vi "Team Member's Favorite Color.vi"(11 "Team Member Name":string) -> (0 "error out":errorcluster, 3 "Favorite Color":u32(colorbox))   [LabVIEW 2024]
uses:
  Team Member/Team Member.lvclass
panel:
  # "Specify your name (i.e. the name of your class) and run the VI. Your favorite color should be displayed."
  # "Note: This VI should require no modification in order to display your favorite color."
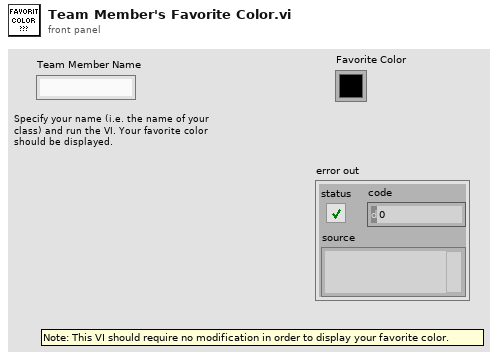
[diagram p1: front panel]
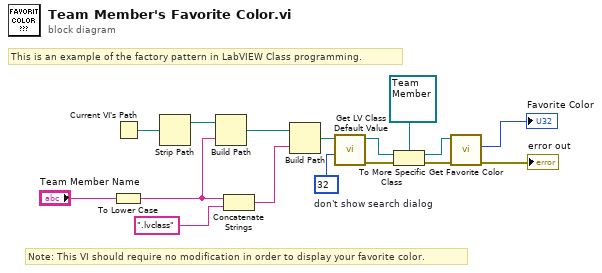
[diagram p0: block diagram]
diagram:
  w1 = u32 32  # don't show search dialog
  # "This is an example of the factory pattern in LabVIEW Class programming."
  # "Note: This VI should require no modification in order to display your favorite color."
  n1 = To Lower Case(string="Team Member Name") -> (all lower case string=w2:string)
  n2 = Current VI's Path() -> (path=w9:path)
  n3 = Strip Path(path=w9) -> (stripped path=w8:path)  [unwired: 1 out]
  n4 = Build Path(base path=w8, name or relative path=w2) -> (appended path=w6:path)
  n5 = Concatenate Strings(w2, ".lvclass" ("string")) -> (w3:string)
  n6 = Build Path(base path=w6, name or relative path=w3) -> (appended path=w7:path)
  n7 = call <vilib>:"Get LV Class Default Value.vi"("options"=w1, "class path"=w7) -> ("error out"=w14:errorcluster, "object"=w13:refnum<class>)  [unwired: 8 in]
  n8 = To More Specific Class(target class=refnum<class "Team Member.lvclass"> refnum ("Team Member"), reference=w13, error in=w14) -> (specific class reference=w11:refnum<class "Team Member.lvclass">, error out=w15:errorcluster)
  n9 = call-dynamic "Get Favorite Color.vi"("error in"=w15, "Team Member in"=w11) -> ("error out"=→"error out":errorcluster, "Favorite Color"=→"Favorite Color":u32)  [unwired: 7 in, 1 out]
